vi "Utility Clean Up Initialize.vi"(0 "VISA session":refnum<visa-resource-name>, 11 "error in (no error)":errorcluster {"code" format="%.0x"}) -> (15 "error out":errorcluster {"code" format="%.0x"})   [LabVIEW 2012, in "Agilent ESG Series.lvlib"]
doc: "This Utility VI closes any open VISA sessions in the event that there is an error during an initialization. It is called only from the hpesgdxx Initialize VI, and is not meant to be altered. Changing this VI can cause the hpesgdxx Initialize VI to operate improperly."
uses:
  Agilent ESG Series.lvlib
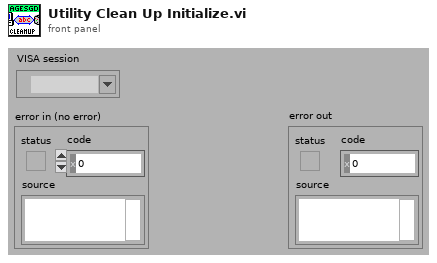
[diagram p1: front panel]
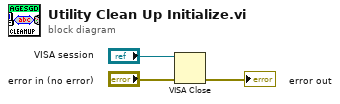
[diagram p0: block diagram]
diagram:
  n1 = VISA Close(VISA resource name="VISA session", error in (no error)="error in (no error)") -> (error out=→"error out":errorcluster)
